vi "CMD Get Graphviz Version.vi"(8 "error in":errorcluster) -> (0 "error out":errorcluster, 3 "Mayor Version":i32)   [LabVIEW 2020, in "SimpleDependencyInspector.lvlib"]
uses:
  Libraries/SimpleDependencyInspector/SimpleDependencyInspector.lvlib
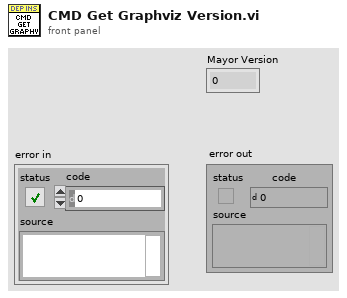
[diagram p1: front panel]
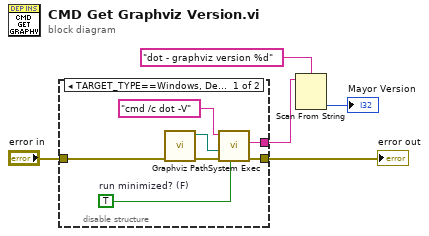
[diagram p0: block diagram]
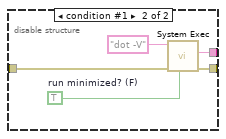
[diagram p2: hidden frame]
diagram:
  n1 = disable-structure shown="TARGET_TYPE==Windows, Default" {
    disable-tunnel: [w11 w17] -> w4
    disable-tunnel: "error in" -> [w10 w16]
    disable-tunnel: [w6 w13] -> w3
    frame condition #0 (active) {
      w9 = TRUE  # run minimized? (F)
      n2 = call "Graphviz Path.vi"("error in"=w10) -> ("error out"=w12:errorcluster, "Graphviz Path"=w8:path)  [unwired: 9 in]
      n3 = call <vilib>:"System Exec.vi"("run minimized? (F)"=w9, "error in (no error)"=w12, "working directory"=w8, "command line"="cmd /c dot -V") -> ("error out"=w11:errorcluster, "standard error"=w6:string)  [unwired: 4 in, 2 out]
    }
    frame condition #1 {
      w15 = TRUE  # run minimized? (F)
      n4 = call <vilib>:"System Exec.vi"("run minimized? (F)"=w15, "error in (no error)"=w16, "command line"="dot -V") -> ("error out"=w17:errorcluster, "standard error"=w13:string)  [unwired: 5 in, 2 out]
    }
  }
  "error out" <- w4
  n5 = Scan From String(format string="dot - graphviz version %d", input string=w3) -> (output 1=→"Mayor Version":i32)  [unwired: 3 in, 3 out]
